vi "HIOKI PW3390 0Adjust.vi"(0 "VISA Resource":refnum<visa-resource-name>, 1 "Set/Query (F: Set)":bool, 11 "error in (no error)":errorcluster, 13 "Error Out (F: Off)":bool) -> (4 "VISA Resource out":refnum<visa-resource-name>, 6 "0Adjust out":enum16{"OK", "BUSY", "ERROR"}(ring), 15 "error out":errorcluster)   [LabVIEW 2009]
doc: "Set/Query\n Set: Execute the zero adjust.\n Query: Query results of the zero adjust.\n\n0Adjust out\n Outputs the query results of the zero adjust.\n\n<B>Note</B>\nThe zero adjust takes more than 30 seconds to execute and in that period, you may get an execution command error."
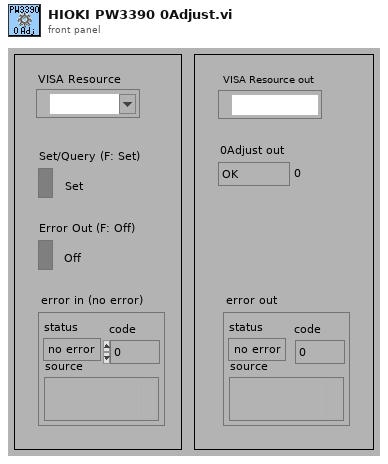
[diagram p1: front panel]
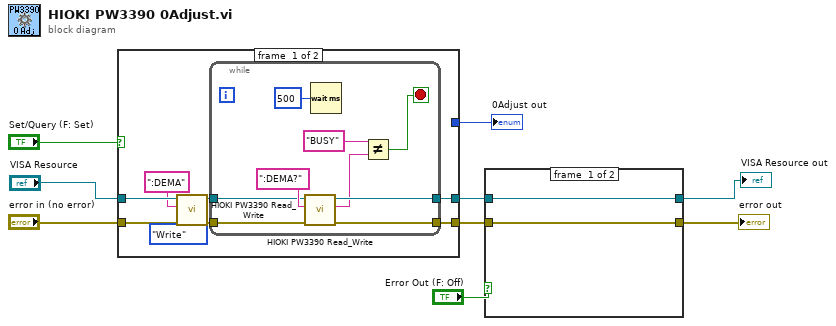
[diagram p0: block diagram]
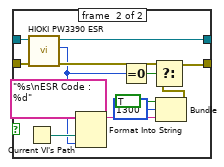
[diagram p2: hidden frame]
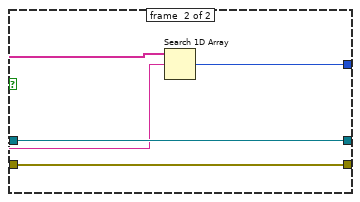
[diagram p3: hidden frame]
diagram:
  n1 = case shown="FALSE" "Set/Query (F: Set)" {
    tunnel: "error in (no error)" -> [w15 w30]
    tunnel: [w12 w33] -> w5
    tunnel: "VISA Resource" -> [w16 w31]
    tunnel: [w13 w32] -> w4
    tunnel: [_ w27] -> w7
    frame #0 {
      n2 = call <instrlib>:"HIOKI PW3390 Read_Write.vi"("Read/Write"=enum16{"Read", "Write"}."Write", "error in (no error)"=w15, "data in"=":DEMA", "VISA Resource"=w16) -> ("error out"=w10:errorcluster, "VISA Resource out"=w11:refnum<visa-resource-name>)  [unwired: 5 in, 1 out]
      n3 = while {
        tunnel: [w24] -> w13
        tunnel: [w23] -> w12
        tunnel: w11 -> [w19]
        tunnel: w10 -> [w18]
        stop <- w22 stop-if-true
        n4 = call <instrlib>:"HIOKI PW3390 Read_Write.vi"("error in (no error)"=w18, "data in"=":DEMA?", "VISA Resource"=w19) -> ("error out"=w23:errorcluster, "data out"=w21:string, "VISA Resource out"=w24:refnum<visa-resource-name>)  [unwired: 6 in]
        n5 = Wait (ms)(milliseconds to wait=u32 500) -> ()  [unwired: 1 out]
        n6 = Not Equal?(x="BUSY", y=w21) -> (x != y?=w22:bool)
      }
    }
    frame #1 {
      n7 = property on="0Adjust out" class="Enum (strict)"() -> ("文字列 []"=w28:string[])  [unwired: 2 in, 2 out]
      n8 = call <instrlib>:"HIOKI PW3390 Read_Write.vi"("error in (no error)"=w30, "data in"=":DEMA?", "VISA Resource"=w31) -> ("error out"=w33:errorcluster, "data out"=w29:string, "VISA Resource out"=w32:refnum<visa-resource-name>)  [unwired: 6 in]
      n9 = Search 1D Array(1D array=w28, element=w29) -> (index of element=w27:i32)  [unwired: 1 in]
    }
  }
  "0Adjust out" <- w7
  n10 = case shown="TRUE" "Error Out (F: Off)" {
    tunnel: w4 -> [w36 w49]
    tunnel: w5 -> [w35 w48]
    tunnel: [w35 w38] -> w3
    tunnel: [w36 w47] -> w1
    frame #0 {
    }
    frame #1 {
      n11 = Current VI's Path() -> (path=w45:path)
      n12 = call <instrlib>:"HIOKI PW3390 ESR.vi"("error in (no error)"=w48, "VISA Resource"=w49) -> ("error out"=w39:errorcluster, "Output Value"=w37:u8, "VISA Resource out"=w47:refnum<visa-resource-name>)  [unwired: 6 in, 1 out]
      n13 = Format Into String(format string="%s\nESR Code : %d", w45, w37) -> (resulting string=w41:string)  [unwired: 2 in, 1 out]
      n14 = Equal To 0?(x=w37) -> (x = 0?=w46:bool)
      n15 = Bundle("status"=TRUE, "code"=1300, w41) -> (w40:cluster{"status":bool, "code":i32, string})  [unwired: 1 in]
      n16 = Select(t=w39, s=w46, f=w40) -> (s? t:f=w38:errorcluster)
    }
  }
  "error out" <- w3
  "VISA Resource out" <- w1
